vi "例7.1.vi"() -> ()   [LabVIEW 2017]
panel:
  out "7（x0=10，dx=2，Y）多条曲线":cluster{i32, i32, cluster{dbl[]}[]}(graph)
  out "6（x0=10，dx=2，Y）多条曲线":cluster{i32, i32, dbl[][]}(graph)
  out "5（x0=10，dx=2，Y）多条曲线":cluster{i32, i32, dbl[]}(graph)
  out "4（x0=10，dx=2，Y）单条曲线":cluster{i32, i32, dbl[]}(graph)
  out "3（Y）多条曲线":cluster{dbl[]}[](graph)
  out "2（Y）多条曲线":dbl[][](graph)
  out "1（Y）单条曲线":dbl[](graph)
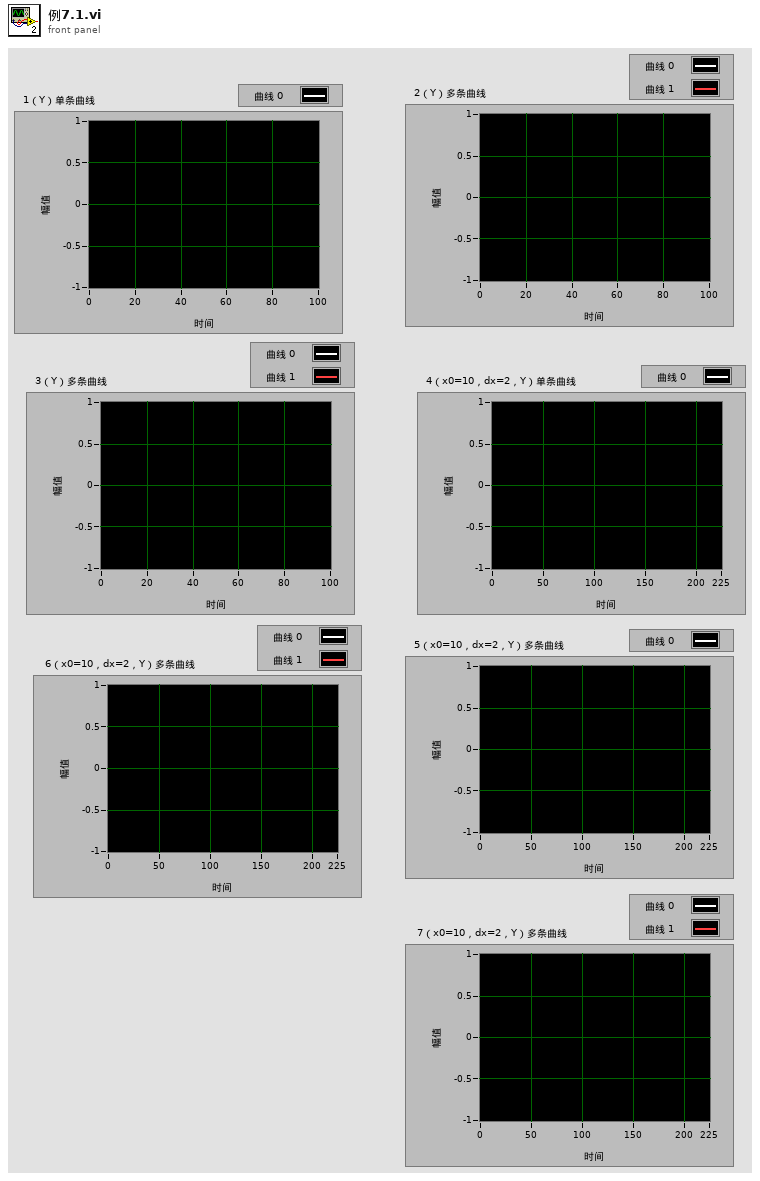
[diagram p1: front panel]
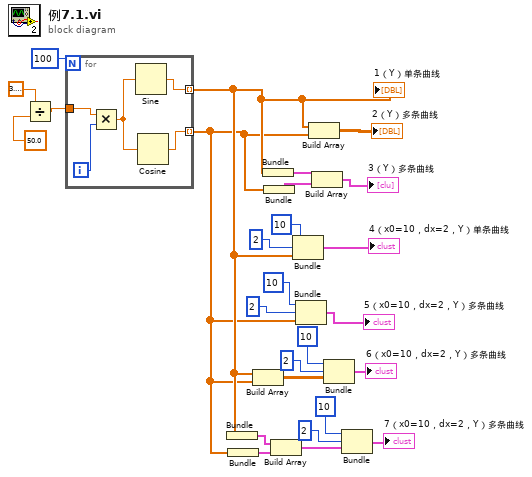
[diagram p0: block diagram]
diagram:
  n1 = Divide(x=3.141592653589793, y=50.0) -> (x/y=w24:dbl)
  n2 = for {
    N: 100 -> [_]
    tunnel: w24 -> [w30]
    tunnel: [w29] -> w4 mode=indexing
    tunnel: [w28] -> w3 mode=indexing
    i -> [w31]
    n3 = Multiply(x=w30, y=w31) -> (x*y=w27:dbl)
    n4 = Sine(x=w27) -> (sin(x)=w29:dbl)
    n5 = Cosine(x=w27) -> (cos(x)=w28:dbl)
  }
  "1（Y）单条曲线" <- w4
  n6 = Bundle(w4) -> (w2:cluster{dbl[]})  [unwired: 1 in]
  n7 = Bundle(w3) -> (w1:cluster{dbl[]})  [unwired: 1 in]
  n8 = Build Array(w4, w3) -> (w12:dbl[][])
  n9 = Bundle(w4) -> (w21:cluster{dbl[]})  [unwired: 1 in]
  n10 = Bundle(w3) -> (w20:cluster{dbl[]})  [unwired: 1 in]
  n11 = Build Array(w2, w1) -> (w8:cluster{dbl[]}[])
  n12 = Bundle(10, 2, w4) -> (→"4（x0=10，dx=2，Y）单条曲线":cluster{i32, i32, dbl[]})  [unwired: 1 in]
  n13 = Bundle(10, 2, w3) -> (→"5（x0=10，dx=2，Y）多条曲线":cluster{i32, i32, dbl[]})  [unwired: 1 in]
  n14 = Build Array(w4, w3) -> (→"2（Y）多条曲线":dbl[][])
  n15 = Build Array(w21, w20) -> (→"3（Y）多条曲线":cluster{dbl[]}[])
  n16 = Bundle(10, 2, w12) -> (→"6（x0=10，dx=2，Y）多条曲线":cluster{i32, i32, dbl[][]})  [unwired: 1 in]
  n17 = Bundle(10, 2, w8) -> (→"7（x0=10，dx=2，Y）多条曲线":cluster{i32, i32, cluster{dbl[]}[]})  [unwired: 1 in]
